vi "close_fw103.vi"(9 "Device reference input":refnum<k24>, 10 "Close signal (bool)":bool) -> ()   [LabVIEW 2020]
uses:
  C:/Users/OPMuser/Documents/labview/fw103/Thorlabs.MotionControl.Controls.dll
  Thorlabs.MotionControl.Controls.dll
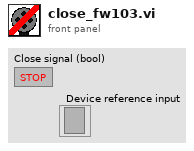
[diagram p1: front panel]
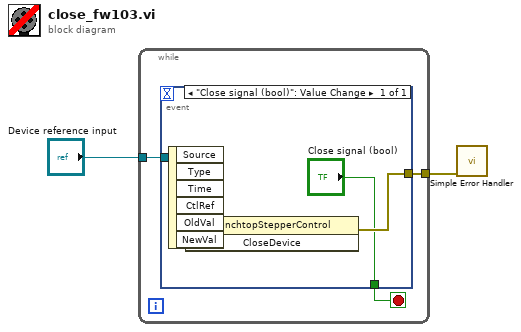
[diagram p0: block diagram]
diagram:
  n1 = while {
    tunnel: "Device reference input" -> [w5]
    tunnel: [w4] -> w1
    stop <- w3 stop-if-true
    n2 = event shown="[0] \"Close signal (bool)\": Value Change" {
      selector: _ -> [_]
      dyn-events: _ -> [_]
      timeout: _ -> [_]
      tunnel: w5 -> [w8]
      tunnel: [w7] -> w4
      tunnel: ["Close signal (bool)"] -> w3
      event "Close signal (bool)": Value Change {
        n3 = event-data() -> ()  [unwired: 1 in, 6 out]
        n4 = invoke class="BenchtopStepperControl" method="CloseDevice"(reference=w8) -> (error out=w7:errorcluster)  [unwired: 2 in, 2 out]
      }
    }
  }
  n5 = call <vilib>:"Simple Error Handler.vi"("error in (no error)"=w1) -> ()  [unwired: 4 in, 5 out]
